vi "Open Data File.vi"(8 "error in (no error)":errorcluster, 9 "Additional parameters":string, 10 "Data Plugin":string="TDM", 11 "File Path":path) -> (0 "error out":errorcluster, 3 "File Ref":refnum<k20>)   [LabVIEW 2015, in "Engine Simulation Toolkit System Explorer.lvlib" / "File Interface.lvlib"]
uses:
  File Interface.lvlib
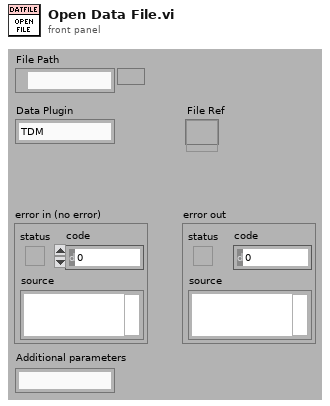
[diagram p1: front panel]
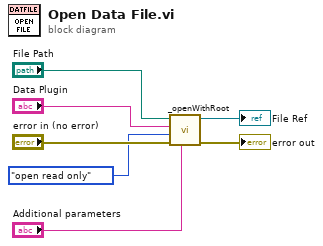
[diagram p0: block diagram]
diagram:
  n1 = call <vilib>:"_openWithRoot.vi"("Additional parameters"="Additional parameters", "error in (no error)"="error in (no error)", "Overwrite Options"=enum16{"create", "open", "open read only"}."open read only", "Storage Type"="Data Plugin", "Storage Location"="File Path") -> ("error out"=→"error out":errorcluster, "Data object"=→"File Ref":refnum<k20>)  [unwired: 5 out]
